vi "Add Entry.vi"(6 "Result":T1, 8 "error in (no error)":errorcluster, 9 "Value":variant, 10 "Name":string, 11 "Results in":refnum<class "Results.lvclass">) -> (0 "error out":errorcluster, 3 "Results out":refnum<class "Results.lvclass">)   [LabVIEW 2020, in "Tester.lvlib" / "Results.lvclass"]
uses:
  Results.lvclass
  Result.ctl
  Entry.ctl
  Results.lvclass/Results.ctl
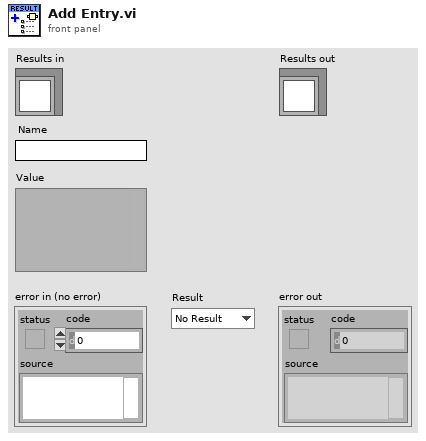
[diagram p1: front panel]
types:
  T1 = typedef "Tester.lvlib/Results.lvclass/Result.ctl" = enum16{"No Result", "Pass", "Fail", "Error", "Abort"}
  T2 = typedef "Tester.lvlib/Results.lvclass/Entry.ctl" = cluster{"Name":string, "Value":variant, "Result":T1}
  T3 = typedef "Tester.lvlib/Results.lvclass/Results Ref.ctl" = cluster{"Entries":T2[], "Overall Result":T1}
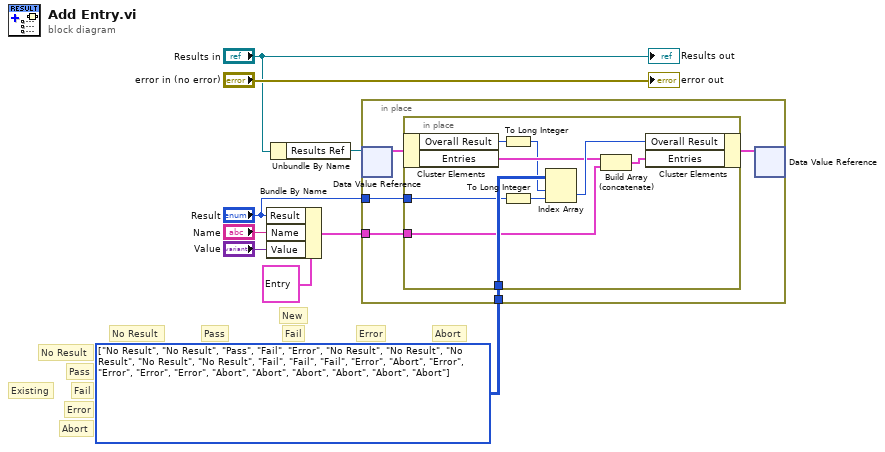
[diagram p0: block diagram]
diagram:
  w1 = T1[][] [[enum."No Result", enum."No Result", enum."Pass", enum."Fail", enum."Error"], [enum."No Result", enum."No Result", enum."No Result", enum."No Result", enum."No Result"], [enum."Fail", enum."Fail", enum."Fail", enum."Error", enum."Abort"], [enum."Error", enum."Error", enum."Error", enum."Error", enum."Abort"], [enum."Abort", enum."Abort", enum."Abort", enum."Abort", enum."Abort"]] items=["No Result", "Pass", "Fail", "Error", "Abort"]
  # "New"
  # "Existing"
  # "Abort"
  # "Abort"
  # "Error"
  # "Error"
  # "Fail"
  # "Fail"
  # "Pass"
  # "Pass"
  # "No Result"
  # "No Result"
  n1 = Bundle By Name(cluster=T2 {"Name"="", "Value"=variant, "Result"=enum."No Result"} ("Entry"), "Result"="Result", "Name"="Name", "Value"="Value") -> (w2:T2)
  n2 = Unbundle By Name("Results in") -> ("Results Ref"=w5:refnum<data-value>)
  n3 = in-place {
    in-place-border: "Result" -> [w12]
    in-place-border: w2 -> [w11]
    in-place-border: w1 -> [w10]
    n4 = in-place-dvr #1(w5) -> (w14:T3)  [unwired: 1 out]
    n5 = in-place {
      in-place-border: w12 -> [w16]
      in-place-border: w11 -> [w19]
      in-place-border: w10 -> [w23]
      n6 = in-place-cluster #2(w14) -> ("Overall Result"=w22:T1, "Entries"=w20:T2[])
      n7 = To Long Integer(number=w22) -> (32bit integer=w17:i32)
      n8 = To Long Integer(number=w16) -> (32bit integer=w15:i32)
      n9 = Index Array(array=w23, index (row)=w17, index (col)=w15) -> (element=w21:T1)
      n10 = Build Array (concatenate)(w20, w19) -> (w18:T2[])
      n11 = in-place-cluster #2("Overall Result"=w21, "Entries"=w18) -> (w13:T3)
    }
    n12 = in-place-dvr #1(w13) -> ()  [unwired: 2 out]
  }
  "error out" <- "error in (no error)"
  "Results out" <- "Results in"
